vi "根据宽和高设定窗口.vi"(8 "错误输入（无错误）":errorcluster, 9 "高":i16, 10 "宽":i16, 11 "引用":refnum<vi>) -> (0 "错误输出":errorcluster, 3 "引用输出":refnum<vi>)   [LabVIEW 8.6, in "窗口操作.lvlib"]
uses:
  <vilib>/Utility/miscctls.llb/LVRectTypeDef.ctl
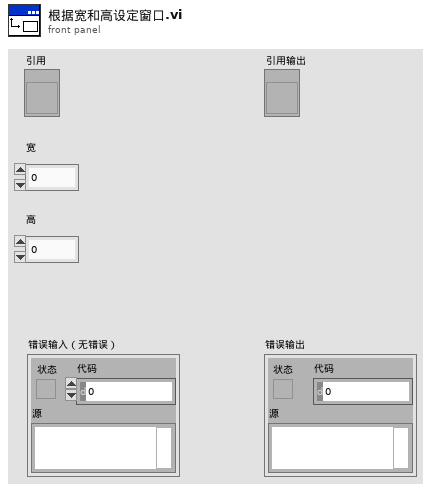
[diagram p1: front panel]
types:
  T1 = typedef "LVRectTypeDef.ctl" = cluster{"Left":i16, "Top":i16, "Right":i16, "Bottom":i16}
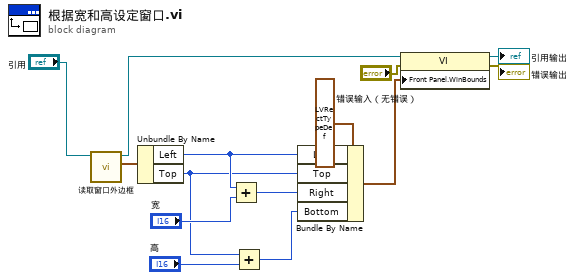
[diagram p0: block diagram]
diagram:
  n1 = call "读取窗口外边框.vi"("引用"="引用") -> ("前面板窗口:窗口边界"=w11:T1, "引用输出"=w1:refnum<vi>)  [unwired: 8 in, 1 out]
  n2 = Unbundle By Name(w11) -> ("Left"=w7:i16, "Top"=w6:i16)
  n3 = Add(x=w7, y="宽") -> (x+y=w5:i16)
  n4 = Add(x=w6, y="高") -> (x+y=w4:i16)
  n5 = Bundle By Name(cluster=T1 ? ("前面板窗口:窗口边界"), "Left"=w7, "Top"=w6, "Right"=w5, "Bottom"=w4) -> (w3:T1)
  n6 = property class="VI"(reference=w1, error in="错误输入（无错误）", "Front Panel.WinBounds"=w3) -> (reference out=→"引用输出":refnum<vi>, error out=→"错误输出":errorcluster)
